vi "IsTransitionCompleteTest.vi"() -> (3 "Were there any errors at all?":bool)   [LabVIEW 2013]
uses:
  Data/TypeDefs/Sailing Regimes.ctl
  Data/TypeDefs/Regime Boundaries.ctl
panel:
  in  "Desired Regime":T1[](array[typedef])
  in  "Current Regime":T1[](array[typedef])
  in  "Last Commanded Regime":T1[](array[typedef])
  out "Actual boolean outputs":bool[](array[boolean])
  in  "Expected boolean outputs":bool[](array[boolean])=[TRUE, TRUE, TRUE, TRUE, TRUE]
  in  "Desired Heading Input":dbl[](array[numeric])=[50.0, 65.0, 170.0, 10.0, 74.0, 0.0]
  in  "Actual Heading Input":dbl[](array[numeric])=[50.0, 50.0, 310.0, 354.0, 69.0, 0.0]
  out "Are chosen regimes right?":bool[](array[boolean])=[TRUE, TRUE, TRUE, TRUE, TRUE]
  # "For the first two tests, the last commanded regime and the desired regime are within 1, so the current regime doesn't matter at all"
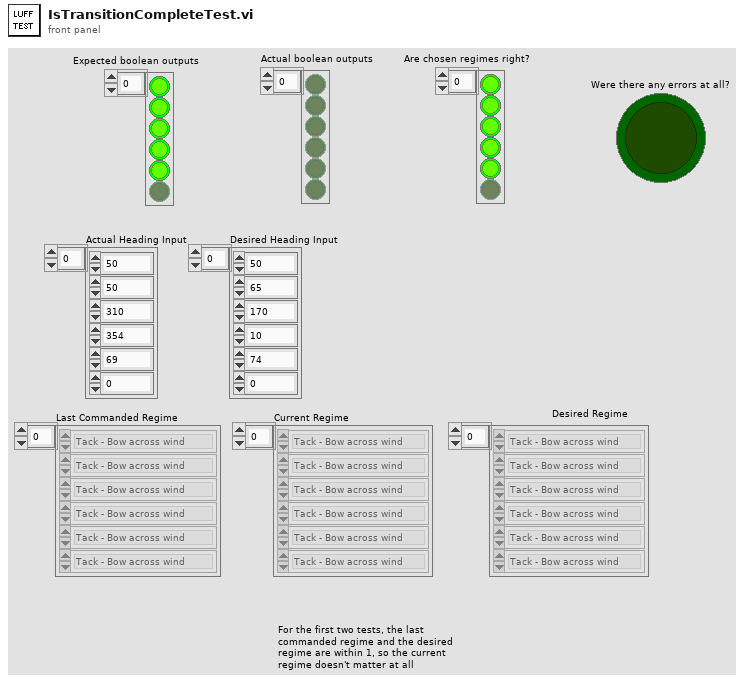
[diagram p1: front panel]
types:
  T1 = typedef "Sailing Regimes.ctl" = enum16{"Tack - Bow across wind", "Upwind - Starboard Tack", "Turn between Upwind/Reach - Starboard Tack", "Reach - Starboard Tack", "Turn between Reach/Run - Starboard Tack", "Run - Starboard Tack", "Jibe - Stern across wind", "Run - Port Tack", "Turn between Reach/Run - Port Tack", "Reach - Port Tack", "Turn between Upwind/Reach - Port Tack", "Upwind - Port Tack"}
  T2 = typedef "Regime Boundaries.ctl" = i32[]
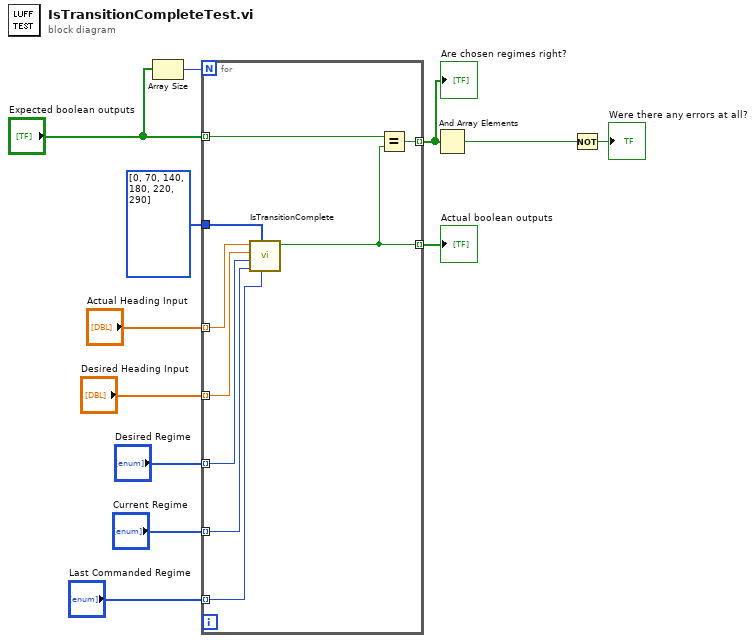
[diagram p0: block diagram]
diagram:
  n1 = Array Size(array="Expected boolean outputs") -> (size(s)=w12:i32)
  n2 = for {
    N: w12 -> [_]
    tunnel: "Expected boolean outputs" -> [w21] mode=indexing
    tunnel: [w20] -> w7 mode=indexing
    tunnel: "Actual Heading Input" -> [w18] mode=indexing
    tunnel: "Desired Heading Input" -> [w17] mode=indexing
    tunnel: [w19] -> w8 mode=indexing
    tunnel: "Last Commanded Regime" -> [w16] mode=indexing
    tunnel: "Desired Regime" -> [w15] mode=indexing
    tunnel: "Current Regime" -> [w14] mode=indexing
    tunnel: T2 [0, 70, 140, 180, 220, 290] ("Default regime boundaries") -> [w13]
    n3 = call "IsTransitionComplete.vi"("Last Commanded Regime"=w16, "Altered regime boundaries"=w13, "Current Regime"=w14, "Desired Regime"=w15, "Desired Heading (deg)"=w17, "Robot Heading (deg)"=w18) -> ("Is Transition Complete?"=w19:bool)  [unwired: 5 in]
    n4 = Equal?(x=w21, y=w19) -> (x = y?=w20:bool)
  }
  "Are chosen regimes right?" <- w7
  "Actual boolean outputs" <- w8
  n5 = And Array Elements(Boolean array=w7) -> (logical AND=w10:bool)
  n6 = Not(x=w10) -> (.not. x?=→"Were there any errors at all?":bool)
